vi "fronts_array.vi"(2 "on":bool[](array[boolean]), 3 "in":bool[](array[boolean])) -> (0 "fall":bool[](array[boolean]), 1 "raise":bool[](array[boolean]))   [LabVIEW 2019, in "Logik.lvlib"]
uses:
  Logik.lvlib
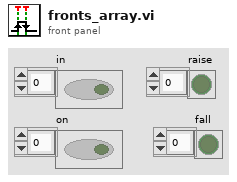
[diagram p1: front panel]
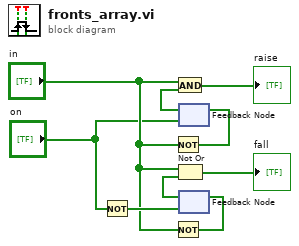
[diagram p0: block diagram]
diagram:
  n1 = Not(x="on") -> (.not. x?=w5:bool[])
  n2 = Not(x="in") -> (.not. x?=w9:bool[])
  n3 = Not(x="in") -> (.not. x?=w7:bool[])
  n4 = feedback #1("on") -> (w8:bool[])
  n5 = And(x="in", y=w8) -> (x .and. y?=→"raise":bool[])
  n6 = feedback-in #1(w9) -> ()
  n7 = feedback #2(w5) -> (w6:bool[])
  n8 = Not Or(1:w6, 2:"in") -> (0:→"fall":bool[])
  n9 = feedback-in #2(w7) -> ()
